vi "GetSingleWfm.vi"(5 "Start Time":timestamp, 6 "error in (no error)":errorcluster, 7 "VISA Refnum in":refnum<visa-resource-name>, 10 "Waveform End":i32=10000, 11 "Channel Name":string) -> (3 "Wfm":waveform(dbl), 4 "error out":errorcluster {"code" format="%.0x"})   [LabVIEW 2011]
uses:
  Desktop/PSDmeasurements2011/Program Files (x86)/National Instruments/LabVIEW 2014/instr.lib/Tektronix TDS 3000 Series/Tektronix TDS 3000 Series.lvlib
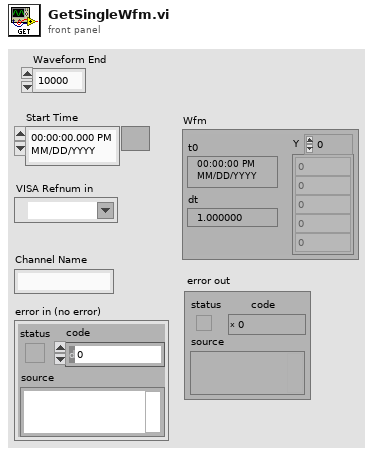
[diagram p1: front panel]
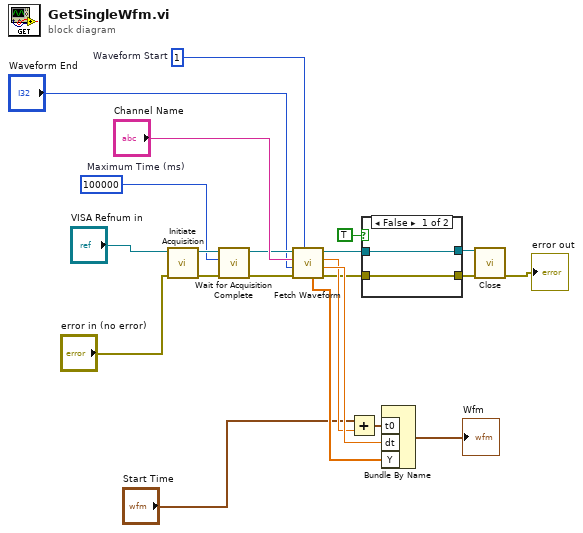
[diagram p0: block diagram]
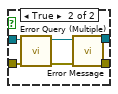
[diagram p2: hidden frame]
diagram:
  w8 = u32 100000  # Maximum Time (ms)
  w7 = 1  # Waveform Start
  n1 = call "Initiate Acquisition.vi"("error in (no error)"="error in (no error)", "VISA Resource Name"="VISA Refnum in") -> ("error out"=w12:errorcluster, "VISA Resource Name Out"=w10:refnum<visa-resource-name>)  [unwired: 8 in]
  n2 = call "Wait for Acquisition Complete.vi"("error in (no error)"=w12, "Maximum Time (10000 ms)"=w8, "VISA Resource Name"=w10) -> ("error out"=w11:errorcluster, "VISA Resource Name Out"=w9:refnum<visa-resource-name>)  [unwired: 7 in]
  n3 = call "Fetch Waveform.vi"("Waveform Start (1)"=w7, "error in (no error)"=w11, "Waveform End (10000)"="Waveform End", "Source (Channel 1)"="Channel Name", "VISA Resource Name"=w9) -> ("error out"=w2:errorcluster, "X Increment"=w17:dbl, "Initial X"=w14:dbl, "VISA Resource Name Out"=w3:refnum<visa-resource-name>, "Waveform Array"=w16:dbl[])  [unwired: 1 in, 1 out]
  n4 = Add(x="Start Time", y=w14) -> (x+y=w13:timestamp)
  n5 = case shown="False" TRUE {
    tunnel: [w23 w30] -> w22
    tunnel: [w24 w29] -> w21
    tunnel: w3 -> [w24 w26]
    tunnel: w2 -> [w23 w25]
    frame False {
    }
    frame True {
      n6 = call "Error Query (Multiple).vi"("error in (no error)"=w25, "VISA Resource Name"=w26) -> ("error out"=w28:errorcluster, "VISA Resource Name Out"=w27:refnum<visa-resource-name>)  [unwired: 6 in, 2 out]
      n7 = call "Error Message.vi"("VISA Resource Name"=w27, "error in (no error)"=w28) -> ("VISA Resource Name Out"=w29:refnum<visa-resource-name>, "error out"=w30:errorcluster)  [unwired: 9 in, 3 out]
    }
  }
  n8 = Bundle By Name("t0"=w13, "dt"=w17, "Y"=w16) -> (→"Wfm":waveform(dbl))  [unwired: 1 in]
  n9 = call "Close.vi"("error in (no error)"=w22, "VISA Resource Name"=w21) -> ("error out"=→"error out":errorcluster)  [unwired: 9 in]
